vi "Matrix_Rotation.vi"(7 "Opt":T1(ring), 11 "Input":dbl[][](array[numeric])) -> (3 "Output":dbl[][](array[numeric]))   [LabVIEW 2014]
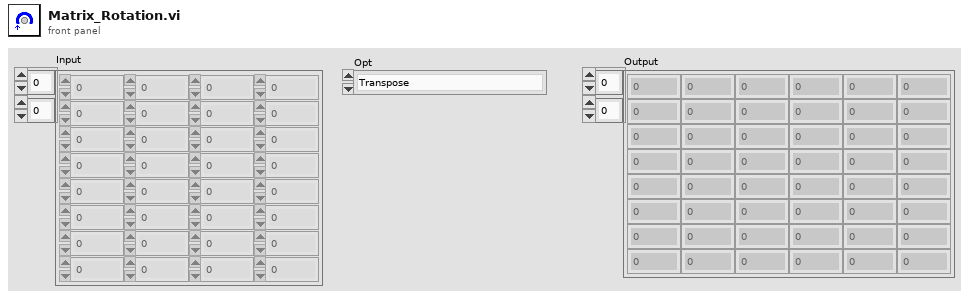
[diagram p1: front panel]
types:
  T1 = enum16{"Transpose", "Vertical Flip", "Horizontal Flip", "Rotate 90", "Rotate 180", "Rotate 270", "Diagonal Flip"}
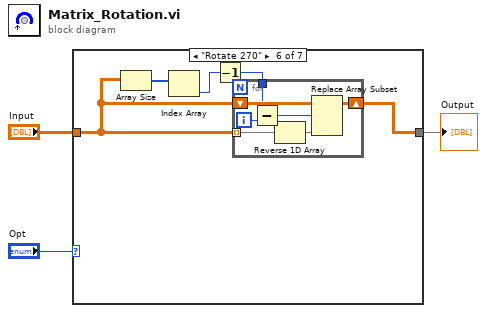
[diagram p0: block diagram]
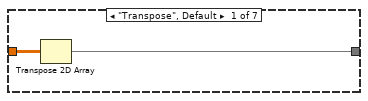
[diagram p2: hidden frame]
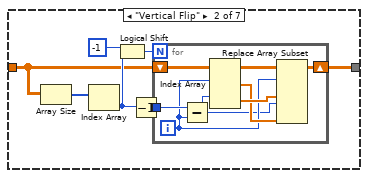
[diagram p3: hidden frame]
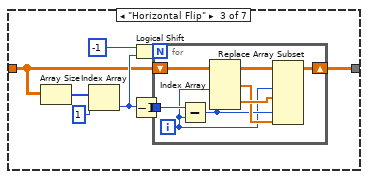
[diagram p4: hidden frame]
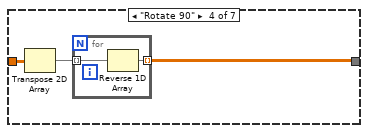
[diagram p5: hidden frame]
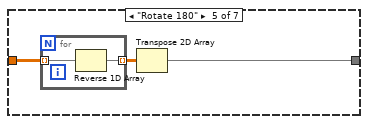
[diagram p6: hidden frame]
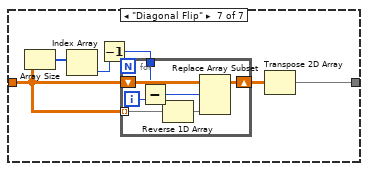
[diagram p7: hidden frame]
diagram:
  n1 = case shown="\"Rotate 270\"" "Opt" {
    tunnel: "Input" -> [w5 w7 w21 w36 w41 w46 w58]
    tunnel: [w4 w6 w20 w35 w40 w45 w57] -> w1
    frame "Transpose", Default {
      n2 = Transpose 2D Array(2D array=w5) -> (transposed array=w4:dbl[][])
    }
    frame "Vertical Flip" {
      n3 = Array Size(array=w7) -> (size(s)=w8:i32[])
      n4 = Index Array(array=w8) -> (element=w10:i32)  [unwired: 1 in]
      n5 = Logical Shift(y=i8 -1, x=w10) -> (x << y=w9:i32)
      n6 = Decrement(x=w10) -> (x-1=w12:i32)
      n7 = for {
        N: w9 -> [_]
        shift-right: [w19] -> w6
        shift-left: w7 -> [w18]
        tunnel: w12 -> [w15]
        i -> [w14]
        n8 = Subtract(x=w15, y=w14) -> (x-y=w13:i32)
        n9 = Index Array(array=w18, index (row) #1=w14, index (row) #2=w13) -> (element #1=w16:dbl[], element #2=w17:dbl[])  [unwired: 2 in]
        n10 = Replace Array Subset(array=w18, new element #1=w17, index (row) #1=w14, new element #2=w16, index (row) #2=w13) -> (w19:dbl[][])  [unwired: 2 in]
      }
    }
    frame "Horizontal Flip" {
      n11 = Array Size(array=w21) -> (size(s)=w26:i32[])
      n12 = Index Array(array=w26, index=1) -> (element=w24:i32)
      n13 = Decrement(x=w24) -> (x-1=w22:i32)
      n14 = Logical Shift(y=i8 -1, x=w24) -> (x << y=w25:i32)
      n15 = for {
        N: w25 -> [_]
        shift-right: [w34] -> w20
        shift-left: w21 -> [w33]
        tunnel: w22 -> [w30]
        i -> [w28]
        n16 = Subtract(x=w30, y=w28) -> (x-y=w29:i32)
        n17 = Index Array(array=w33, index (col) #1=w28, index (col) #2=w29) -> (element #1=w31:dbl[], element #2=w32:dbl[])  [unwired: 2 in]
        n18 = Replace Array Subset(array=w33, new element #1=w32, index (col) #1=w28, new element #2=w31, index (col) #2=w29) -> (w34:dbl[][])  [unwired: 2 in]
      }
    }
    frame "Rotate 90" {
      n19 = Transpose 2D Array(2D array=w36) -> (transposed array=w37:dbl[][])
      n20 = for {
        tunnel: w37 -> [w39] mode=indexing
        tunnel: [w38] -> w35 mode=indexing
        n21 = Reverse 1D Array(array=w39) -> (reversed array=w38:dbl[])
      }
    }
    frame "Rotate 180" {
      n22 = for {
        tunnel: w41 -> [w44] mode=indexing
        tunnel: [w43] -> w42 mode=indexing
        n23 = Reverse 1D Array(array=w44) -> (reversed array=w43:dbl[])
      }
      n24 = Transpose 2D Array(2D array=w42) -> (transposed array=w40:dbl[][])
    }
    frame "Rotate 270" {
      n25 = Array Size(array=w46) -> (size(s)=w47:i32[])
      n26 = Index Array(array=w47) -> (element=w49:i32)  [unwired: 1 in]
      n27 = Decrement(x=w49) -> (x-1=w48:i32)
      n28 = for {
        shift-right: [w56] -> w45
        shift-left: w46 -> [w55]
        tunnel: w48 -> [w53]
        tunnel: w46 -> [w50] mode=indexing
        i -> [w54]
        n29 = Subtract(x=w53, y=w54) -> (x-y=w52:i32)
        n30 = Reverse 1D Array(array=w50) -> (reversed array=w51:dbl[])
        n31 = Replace Array Subset(array=w55, new element=w51, index (row)=w52) -> (w56:dbl[][])  [unwired: 1 in]
      }
    }
    frame "Diagonal Flip" {
      n32 = Array Size(array=w58) -> (size(s)=w60:i32[])
      n33 = Index Array(array=w60) -> (element=w62:i32)  [unwired: 1 in]
      n34 = Decrement(x=w62) -> (x-1=w61:i32)
      n35 = for {
        shift-right: [w69] -> w59
        shift-left: w58 -> [w68]
        tunnel: w61 -> [w66]
        tunnel: w58 -> [w63] mode=indexing
        i -> [w67]
        n36 = Subtract(x=w66, y=w67) -> (x-y=w65:i32)
        n37 = Reverse 1D Array(array=w63) -> (reversed array=w64:dbl[])
        n38 = Replace Array Subset(array=w68, new element=w64, index (row)=w65) -> (w69:dbl[][])  [unwired: 1 in]
      }
      n39 = Transpose 2D Array(2D array=w59) -> (transposed array=w57:dbl[][])
    }
  }
  "Output" <- w1
